vi "svfa_Conversion Utility (spectrum info).vi"(4 "spectral density desired":T1(ring), 5 "dx":dbl format="%.2f", 6 "desired scaling":T8 {"dB reference (0: no change)" format="%.2f"}, 7 "x0":dbl format="%.2f", 8 "error in (no error)":errorcluster, 10 "spectrum info in":T2={"channel name"="", "description"="", "x-axis units"=0, "spectral info"={"spectrum type"=enum."Power [Magnitude^2]", "linear/dB"=enum."linear", "window"=0, "window size"=0, "FFT size"=0}, "engineering units"=1, "custom label"="", "dB reference [EU]"=0.0, "peak units"=enum."rms", "weighting filter"=0, "spectral density?"=FALSE, "unit label"="", "spectrum skewed?"=FALSE, "complimentary spectrum units"=enum."none"} {"x-axis units" items=["Time (s)"=0, "Frequency-CB (Hz)"=1, "Frequency-CPB (Hz)"=1248, "Frequency-Arbitrary (Hz)"=2357, "Quefrency (s)"=2, "Revolutions (rev)"=3, "Order"=4, "Speed (RPM)"=11, "Speed (rad/s)"=21, "Index"=65535]; "weighting filter" items=["Linear", "A-weighting", "B-weighting", "C-weighting", "ITU-R 468-4", "Dolby", "CCITT", "C-message", "Wb", "Wc", "Wd", "We", "Wf", "Wh", "Wj", "Wk", "Wm", "AES17 20 kHz lowpass", "AES17 40 kHz lowpass", "AES17 20 kHz highpass", "AES17 40 kHz highpass"]; "dB reference [EU]" format="%.2f"; "engineering units" items=["custom..."=0, "V"=1, "A"=21, "C"=30, "pC"=31, "s"=32, "-"=29, "Pa"=2, "N"=20, "g"=3, "m/s^2"=4, "m/s"=5, "m"=6, "mm/s"=12, "mm"=13, "micron/s"=14, "micron"=15, "in/s^2"=7, "in/s"=8, "in"=9, "mil/s"=10, "mil"=11, "rad/s^2"=16, "rad/s"=17, "rad"=18, "deg/s^2"=26, "deg/s"=27, "deg"=28, "RPM"=22, "cycle/s^2"=23, "Hz"=24, "cycle"=25, "strain"=19]; "spectral info"."window" items=["None "=0, "Hanning"=1, "Hamming"=2, "Blackman-Harris"=3, "Exact Blackman"=4, "Blackman"=5, "Flat Top"=6, "4 Term B-Harris "=7, "7 Term B-Harris"=8, "Low Sidelobe"=9, "Force - Exponential"=10, "Gaussian"=62]}, 11 "input signal":dbl[](array[numeric]) format="%.2f") -> (0 "error out":errorcluster, 2 "spectrum info out":T2={"channel name"="", "description"="", "x-axis units"=0, "spectral info"={"spectrum type"=enum."Power [Magnitude^2]", "linear/dB"=enum."linear", "window"=0, "window size"=0, "FFT size"=0}, "engineering units"=1, "custom label"="", "dB reference [EU]"=0.0, "peak units"=enum."rms", "weighting filter"=0, "spectral density?"=FALSE, "unit label"="", "spectrum skewed?"=FALSE, "complimentary spectrum units"=enum."none"} {"x-axis units" items=["Time (s)"=0, "Frequency-CB (Hz)"=1, "Frequency-CPB (Hz)"=1248, "Frequency-Arbitrary (Hz)"=2357, "Quefrency (s)"=2, "Revolutions (rev)"=3, "Order"=4, "Speed (RPM)"=11, "Speed (rad/s)"=21, "Index"=65535]; "weighting filter" items=["Linear", "A-weighting", "B-weighting", "C-weighting", "ITU-R 468-4", "Dolby", "CCITT", "C-message", "Wb", "Wc", "Wd", "We", "Wf", "Wh", "Wj", "Wk", "Wm", "AES17 20 kHz lowpass", "AES17 40 kHz lowpass", "AES17 20 kHz highpass", "AES17 40 kHz highpass"]; "dB reference [EU]" format="%.2f"; "engineering units" items=["custom..."=0, "V"=1, "A"=21, "C"=30, "pC"=31, "s"=32, "-"=29, "Pa"=2, "N"=20, "g"=3, "m/s^2"=4, "m/s"=5, "m"=6, "mm/s"=12, "mm"=13, "micron/s"=14, "micron"=15, "in/s^2"=7, "in/s"=8, "in"=9, "mil/s"=10, "mil"=11, "rad/s^2"=16, "rad/s"=17, "rad"=18, "deg/s^2"=26, "deg/s"=27, "deg"=28, "RPM"=22, "cycle/s^2"=23, "Hz"=24, "cycle"=25, "strain"=19]; "spectral info"."window" items=["None "=0, "Hanning"=1, "Hamming"=2, "Blackman-Harris"=3, "Exact Blackman"=4, "Blackman"=5, "Flat Top"=6, "4 Term B-Harris "=7, "7 Term B-Harris"=8, "Low Sidelobe"=9, "Force - Exponential"=10, "Gaussian"=62]}, 3 "converted signal":dbl[](array[numeric]) format="%.2f")   [LabVIEW 2017]
uses:
  <vilib>/addons/_NISVFA/_Shared subVIs/Controls/svc_Spectrum Info.ctl
  <vilib>/addons/_NISVFA/_Shared subVIs/Controls/svc_X-Axis Units.ctl
  <vilib>/addons/_NISVFA/_Shared subVIs/Controls/svc_Spectrum Type.ctl
  <vilib>/addons/_NISVFA/_Shared subVIs/Controls/svc_Engineering Units Text Ring.ctl
  <vilib>/addons/_NISVFA/_Shared subVIs/Controls/svc_Weighting Filter Text Ring.ctl
  <vilib>/addons/_NISVFA/_Shared subVIs/Controls/svc_Complimentary Spectrum Units.ctl
  <vilib>/addons/_NISVFA/_Shared subVIs/Common/svc_Window Parameters.vi
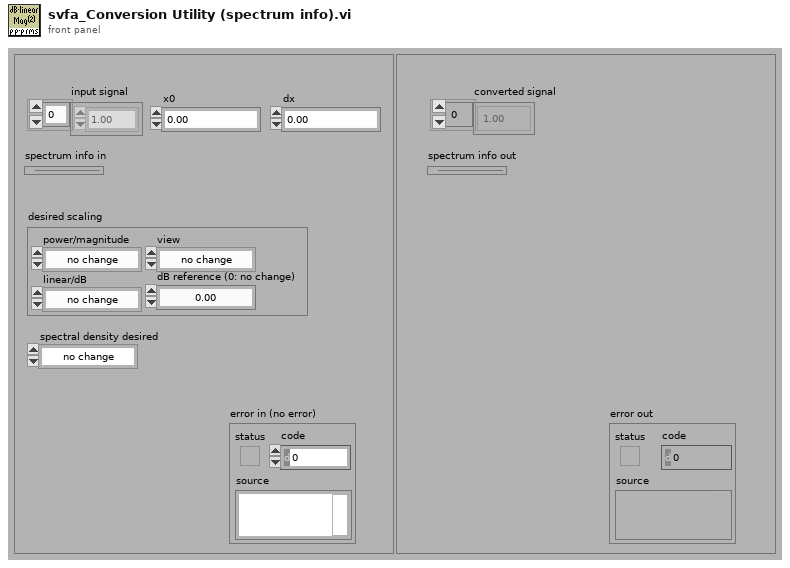
[diagram p1: front panel]
types:
  T1 = enum16{"no change", "spectrum", "spectral density"}
  T2 = typedef "svc_Spectrum Info.ctl" = cluster{"channel name":string, "description":string, "x-axis units":T3, "spectral info":cluster{"spectrum type":T4, "linear/dB":enum16{"linear", "dB"}, "window":u16, "window size":i32, "FFT size":i32}, "engineering units":T5, "custom label":string, "dB reference [EU]":dbl, "peak units":enum16{"rms", "peak", "peak-peak"}, "weighting filter":T6, "spectral density?":bool, "unit label":string, "spectrum skewed?":bool, "complimentary spectrum units":T7}
  T3 = typedef "svc_X-Axis Units.ctl" = u16
  T4 = typedef "svc_Spectrum Type.ctl" = enum16{"FFT Spectrum [complex]", "Amplitude [Magnitude]", "Power [Magnitude^2]", "Cross Spectrum [complex]", "Frequency Response [Complex]"}
  T5 = typedef "svc_Engineering Units Text Ring.ctl" = u16
  T6 = typedef "svc_Weighting Filter Text Ring.ctl" = u16
  T7 = typedef "svc_Complimentary Spectrum Units.ctl" = enum16{"none", "radians", "degrees", "cycles", "imaginary"}
  T8 = cluster{"linear/dB":enum16{"no change", "linear", "dB"}, "dB reference (0: no change)":dbl, "power/magnitude":enum16{"no change", "power", "magnitude"}, "view":enum16{"no change", "rms", "peak", "peak-peak"}}
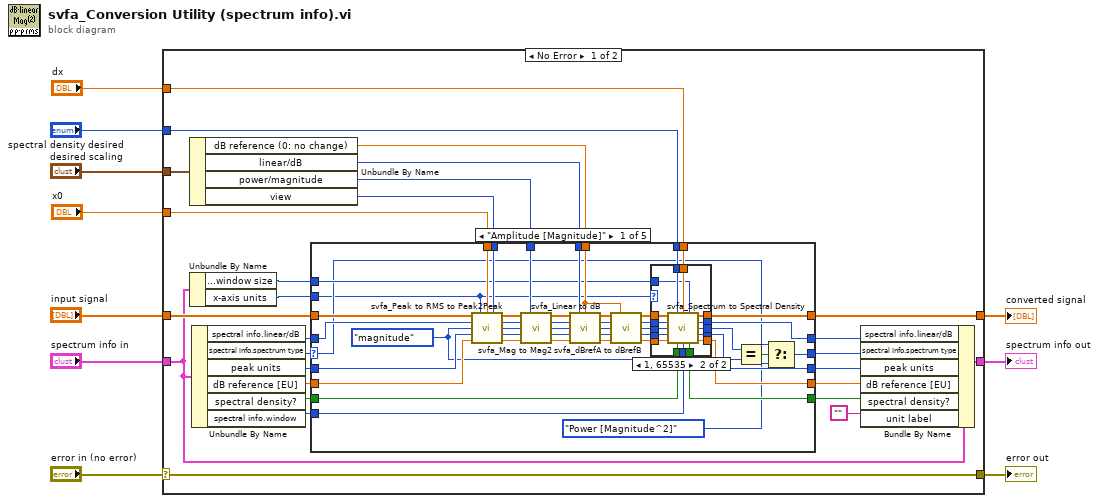
[diagram p0: block diagram]
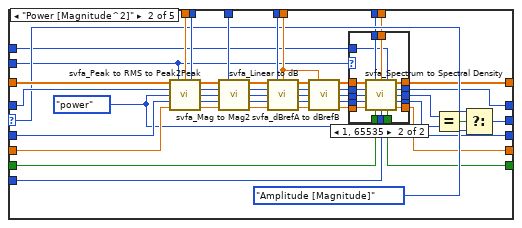
[diagram p3: hidden frame]
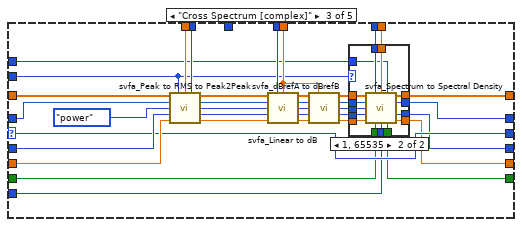
[diagram p5: hidden frame]
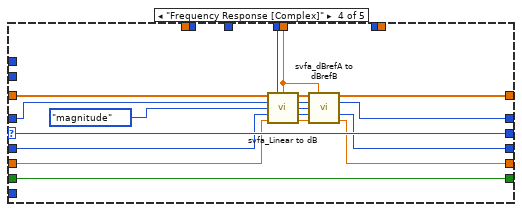
[diagram p7: hidden frame]
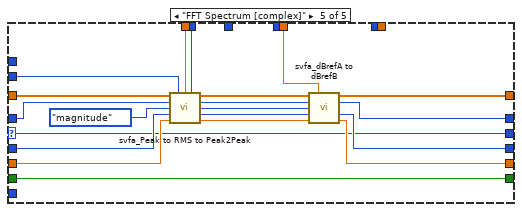
[diagram p8: hidden frame]
diagram:
  n1 = case shown="No Error" "error in (no error)" {
    selector: "error in (no error)" -> [w36 w268]
    tunnel: "input signal" -> [w33 w270]
    tunnel: [w20 w270] -> w4
    tunnel: "desired scaling" -> [w37 _]
    tunnel: "spectrum info in" -> [w16 w269]
    tunnel: [w26 w269] -> w7
    tunnel: [w36 w268] -> w5
    tunnel: "x0" -> [w31 _]
    tunnel: "spectral density desired" -> [w25 _]
    tunnel: "dx" -> [w24 _]
    frame No Error {
      n2 = Unbundle By Name(w37) -> ("dB reference (0: no change)"=w30:dbl, "linear/dB"=w35:enum16{"no change", "linear", "dB"}, "power/magnitude"=w34:enum16{"no change", "power", "magnitude"}, "view"=w32:enum16{"no change", "rms", "peak", "peak-peak"})
      n3 = Unbundle By Name(w16) -> ("spectral info.window size"=w14:i32, "x-axis units"=w15:T3)
      n4 = Unbundle By Name(w16) -> ("spectral info.linear/dB"=w28:enum16{"linear", "dB"}, "spectral info.spectrum type"=w12:T4, "peak units"=w13:enum16{"rms", "peak", "peak-peak"}, "dB reference [EU]"=w29:dbl, "spectral density?"=w23:bool, "spectral info.window"=w22:u16)
      n5 = case shown="\"Amplitude [Magnitude]\"" w12 {
        selector: w12 -> [w40 w124 w190 w240 w248]
        tunnel: w35 -> [w83 w151 w209 w247 _]
        tunnel: w34 -> [w82 w150 _ _ _]
        tunnel: w33 -> [w81 w149 w208 w237 w267]
        tunnel: w32 -> [w77 w145 w206 _ w266]
        tunnel: w31 -> [w67 w135 w202 _ w265]
        tunnel: w30 -> [w64 w132 w201 w242 w264]
        tunnel: w29 -> [w62 w130 w199 w234 w263]
        tunnel: w28 -> [w61 w129 w198 w236 w262]
        tunnel: [w59 w127 w190 w240 w248] -> w27
        tunnel: w25 -> [w58 w107 w186 _ _]
        tunnel: w24 -> [w57 w106 w185 _ _]
        tunnel: w23 -> [w56 w114 w176 w232 w251]
        tunnel: w22 -> [w55 w113 w175 _ _]
        tunnel: [w54 w112 w174 w232 w251] -> w21
        tunnel: [w48 w122 w177 w239 w253] -> w20
        tunnel: [w47 w108 w178 w238 w252] -> w19
        tunnel: [w46 w110 w179 w230 w249] -> w18
        tunnel: [w45 w109 w180 w233 w250] -> w17
        tunnel: w15 -> [w38 w121 w187 _ w261]
        tunnel: w14 -> [w44 w120 w188 _ _]
        tunnel: w13 -> [w43 w126 w197 w231 w260]
        frame "Amplitude [Magnitude]" {
          w42 = enum16{"power", "magnitude"}."magnitude" ("power/magnitude")
          n6 = call <vilib>:"svfa_Peak to RMS to Peak2Peak.vi"("input signal"=w81, "x-axis units"=w38, "x0"=w67, "view desired"=w77, "linear/dB"=w61, "power/magnitude"=w42, "view in"=w43, "dB reference"=w62) -> ("scale converted signal"=w80:dbl[], "linear/dB (dupl)"=w76:enum16{"linear", "dB"}, "power/magnitude (dupl)"=w66:enum16{"power", "magnitude"}, "view out"=w73:enum16{"rms", "peak", "peak-peak"}, "dB reference (dupl)"=w72:dbl)  [unwired: 3 in]
          n7 = call <vilib>:"svfa_Mag to Mag2.vi"("input signal"=w80, "power/magnitude desired"=w82, "linear/dB"=w76, "power/magnitude"=w66, "view"=w73, "dB reference"=w72) -> ("converted signal"=w79:dbl[], "dup linear/dB"=w75:enum16{"linear", "dB"}, "power/magnitude (out)"=w65:enum16{"power", "magnitude"}, "dup view"=w70:enum16{"rms", "peak", "peak-peak"}, "dB reference (out)"=w71:dbl)  [unwired: 5 in]
          n8 = call <vilib>:"svfa_Linear to dB.vi"("input signal"=w79, "linear/dB desired"=w83, "dB reference (desired)"=w64, "linear/dB (in)"=w75, "power/magnitude"=w65, "view in"=w70, "dB reference"=w71) -> ("converted signal"=w78:dbl[], "linear/dB (out)"=w74:enum16{"linear", "dB"}, "power/magnitude (dupl)"=w63:enum16{"power", "magnitude"}, "view out"=w69:enum16{"rms", "peak", "peak-peak"}, "dB reference (dupl)"=w68:dbl)  [unwired: 4 in]
          n9 = call <vilib>:"svfa_dBrefA to dBrefB.vi"("input signal"=w78, "dB reference (desired)"=w64, "linear/dB"=w74, "power/magnitude"=w63, "view"=w69, "dB reference"=w68) -> ("converted signal"=w49:dbl[], "linear/dB (dupl)"=w50:enum16{"linear", "dB"}, "power/magnitude (dupl)"=w51:enum16{"power", "magnitude"}, "dup view"=w52:enum16{"rms", "peak", "peak-peak"}, "dB reference (out)"=w53:dbl)  [unwired: 5 in]
          n10 = case shown="1, 65535" w38 {
            tunnel: w58 -> [_ w105]
            tunnel: w57 -> [_ w104]
            tunnel: w56 -> [w84 w103]
            tunnel: w55 -> [_ w102]
            tunnel: [w84 w101] -> w54
            tunnel: w53 -> [w85 w100]
            tunnel: w52 -> [w86 w99]
            tunnel: w51 -> [w87 w98]
            tunnel: w50 -> [w88 w97]
            tunnel: w49 -> [w89 w96]
            tunnel: [w89 w95] -> w48
            tunnel: [w88 w94] -> w47
            tunnel: [w86 w93] -> w46
            tunnel: [w85 w92] -> w45
            tunnel: w44 -> [_ w91]
            tunnel: [w87 w90] -> w41
            frame Default {
            }
            frame 1, 65535 {
              n11 = call <vilib>:"svfa_Spectrum to Spectral Density.vi"("input signal"=w96, "spectral density desired"=w105, "df"=w104, "window size"=w91, "linear/dB"=w97, "power/magnitude"=w98, "view"=w99, "dB reference"=w100, "spectral density?"=w103, "window"=w102) -> ("converted signal"=w95:dbl[], "dup linear/dB"=w94:enum16{"linear", "dB"}, "power/magnitude (dupl)"=w90:enum16{"power", "magnitude"}, "dup view"=w93:enum16{"rms", "peak", "peak-peak"}, "spectral density?"=w101:bool, "dB reference (out)"=w92:dbl)
            }
          }
          n12 = Equal?(x=w41, y=w42) -> (x = y?=w60:bool)
          n13 = Select(t=w40, s=w60, f=svc_Spectrum_Type."Power [Magnitude^2]" ("spectral info.spectrum type")) -> (s? t:f=w59:T4)
        }
        frame "Power [Magnitude^2]" {
          w125 = enum16{"power", "magnitude"}."power" ("power/magnitude")
          n14 = call <vilib>:"svfa_Peak to RMS to Peak2Peak.vi"("input signal"=w149, "x-axis units"=w121, "x0"=w135, "view desired"=w145, "linear/dB"=w129, "power/magnitude"=w125, "view in"=w126, "dB reference"=w130) -> ("scale converted signal"=w148:dbl[], "linear/dB (dupl)"=w144:enum16{"linear", "dB"}, "power/magnitude (dupl)"=w134:enum16{"power", "magnitude"}, "view out"=w141:enum16{"rms", "peak", "peak-peak"}, "dB reference (dupl)"=w140:dbl)  [unwired: 3 in]
          n15 = call <vilib>:"svfa_Mag to Mag2.vi"("input signal"=w148, "power/magnitude desired"=w150, "linear/dB"=w144, "power/magnitude"=w134, "view"=w141, "dB reference"=w140) -> ("converted signal"=w147:dbl[], "dup linear/dB"=w143:enum16{"linear", "dB"}, "power/magnitude (out)"=w133:enum16{"power", "magnitude"}, "dup view"=w138:enum16{"rms", "peak", "peak-peak"}, "dB reference (out)"=w139:dbl)  [unwired: 5 in]
          n16 = call <vilib>:"svfa_Linear to dB.vi"("input signal"=w147, "linear/dB desired"=w151, "dB reference (desired)"=w132, "linear/dB (in)"=w143, "power/magnitude"=w133, "view in"=w138, "dB reference"=w139) -> ("converted signal"=w146:dbl[], "linear/dB (out)"=w142:enum16{"linear", "dB"}, "power/magnitude (dupl)"=w131:enum16{"power", "magnitude"}, "view out"=w137:enum16{"rms", "peak", "peak-peak"}, "dB reference (dupl)"=w136:dbl)  [unwired: 4 in]
          n17 = call <vilib>:"svfa_dBrefA to dBrefB.vi"("input signal"=w146, "dB reference (desired)"=w132, "linear/dB"=w142, "power/magnitude"=w131, "view"=w137, "dB reference"=w136) -> ("converted signal"=w119:dbl[], "linear/dB (dupl)"=w118:enum16{"linear", "dB"}, "power/magnitude (dupl)"=w117:enum16{"power", "magnitude"}, "dup view"=w116:enum16{"rms", "peak", "peak-peak"}, "dB reference (out)"=w115:dbl)  [unwired: 5 in]
          n18 = case shown="1, 65535" w121 {
            tunnel: w107 -> [_ w173]
            tunnel: w106 -> [_ w172]
            tunnel: w114 -> [w152 w171]
            tunnel: w113 -> [_ w170]
            tunnel: [w152 w169] -> w112
            tunnel: w115 -> [w153 w168]
            tunnel: w116 -> [w154 w167]
            tunnel: w117 -> [w155 w166]
            tunnel: w118 -> [w156 w165]
            tunnel: w119 -> [w157 w164]
            tunnel: [w157 w163] -> w122
            tunnel: [w156 w162] -> w108
            tunnel: [w154 w161] -> w110
            tunnel: [w153 w160] -> w109
            tunnel: w120 -> [_ w159]
            tunnel: [w155 w158] -> w111
            frame Default {
            }
            frame 1, 65535 {
              n19 = call <vilib>:"svfa_Spectrum to Spectral Density.vi"("input signal"=w164, "spectral density desired"=w173, "df"=w172, "window size"=w159, "linear/dB"=w165, "power/magnitude"=w166, "view"=w167, "dB reference"=w168, "spectral density?"=w171, "window"=w170) -> ("converted signal"=w163:dbl[], "dup linear/dB"=w162:enum16{"linear", "dB"}, "power/magnitude (dupl)"=w158:enum16{"power", "magnitude"}, "dup view"=w161:enum16{"rms", "peak", "peak-peak"}, "spectral density?"=w169:bool, "dB reference (out)"=w160:dbl)
            }
          }
          n20 = Equal?(x=w111, y=w125) -> (x = y?=w128:bool)
          n21 = Select(t=w124, s=w128, f=svc_Spectrum_Type."Amplitude [Magnitude]" ("spectral info.spectrum type")) -> (s? t:f=w127:T4)
        }
        frame "Cross Spectrum [complex]" {
          n22 = call <vilib>:"svfa_Peak to RMS to Peak2Peak.vi"("input signal"=w208, "x-axis units"=w187, "x0"=w202, "view desired"=w206, "linear/dB"=w198, "power/magnitude"=enum16{"power", "magnitude"}."power", "view in"=w197, "dB reference"=w199) -> ("scale converted signal"=w195:dbl[], "linear/dB (dupl)"=w194:enum16{"linear", "dB"}, "power/magnitude (dupl)"=w193:enum16{"power", "magnitude"}, "view out"=w192:enum16{"rms", "peak", "peak-peak"}, "dB reference (dupl)"=w191:dbl)  [unwired: 3 in]
          n23 = call <vilib>:"svfa_Linear to dB.vi"("input signal"=w195, "linear/dB desired"=w209, "dB reference (desired)"=w201, "linear/dB (in)"=w194, "power/magnitude"=w193, "view in"=w192, "dB reference"=w191) -> ("converted signal"=w207:dbl[], "linear/dB (out)"=w205:enum16{"linear", "dB"}, "power/magnitude (dupl)"=w200:enum16{"power", "magnitude"}, "view out"=w204:enum16{"rms", "peak", "peak-peak"}, "dB reference (dupl)"=w203:dbl)  [unwired: 4 in]
          n24 = call <vilib>:"svfa_dBrefA to dBrefB.vi"("input signal"=w207, "dB reference (desired)"=w201, "linear/dB"=w205, "power/magnitude"=w200, "view"=w204, "dB reference"=w203) -> ("converted signal"=w189:dbl[], "linear/dB (dupl)"=w184:enum16{"linear", "dB"}, "power/magnitude (dupl)"=w183:enum16{"power", "magnitude"}, "dup view"=w182:enum16{"rms", "peak", "peak-peak"}, "dB reference (out)"=w181:dbl)  [unwired: 5 in]
          n25 = case shown="1, 65535" w187 {
            tunnel: w186 -> [_ w229]
            tunnel: w185 -> [_ w228]
            tunnel: w176 -> [w210 w227]
            tunnel: w175 -> [_ w226]
            tunnel: [w210 w225] -> w174
            tunnel: w181 -> [w211 w224]
            tunnel: w182 -> [w212 w223]
            tunnel: w183 -> [_ w222]
            tunnel: w184 -> [w213 w221]
            tunnel: w189 -> [w214 w220]
            tunnel: [w214 w219] -> w177
            tunnel: [w213 w218] -> w178
            tunnel: [w212 w217] -> w179
            tunnel: [w211 w216] -> w180
            tunnel: w188 -> [_ w215]
            frame Default {
            }
            frame 1, 65535 {
              n26 = call <vilib>:"svfa_Spectrum to Spectral Density.vi"("input signal"=w220, "spectral density desired"=w229, "df"=w228, "window size"=w215, "linear/dB"=w221, "power/magnitude"=w222, "view"=w223, "dB reference"=w224, "spectral density?"=w227, "window"=w226) -> ("converted signal"=w219:dbl[], "dup linear/dB"=w218:enum16{"linear", "dB"}, "dup view"=w217:enum16{"rms", "peak", "peak-peak"}, "spectral density?"=w225:bool, "dB reference (out)"=w216:dbl)  [unwired: 1 out]
            }
          }
        }
        frame "Frequency Response [Complex]" {
          n27 = call <vilib>:"svfa_Linear to dB.vi"("input signal"=w237, "linear/dB desired"=w247, "dB reference (desired)"=w242, "linear/dB (in)"=w236, "power/magnitude"=enum16{"power", "magnitude"}."magnitude", "view in"=w231, "dB reference"=w234) -> ("converted signal"=w246:dbl[], "linear/dB (out)"=w245:enum16{"linear", "dB"}, "power/magnitude (dupl)"=w241:enum16{"power", "magnitude"}, "view out"=w244:enum16{"rms", "peak", "peak-peak"}, "dB reference (dupl)"=w243:dbl)  [unwired: 4 in]
          n28 = call <vilib>:"svfa_dBrefA to dBrefB.vi"("input signal"=w246, "dB reference (desired)"=w242, "linear/dB"=w245, "power/magnitude"=w241, "view"=w244, "dB reference"=w243) -> ("converted signal"=w239:dbl[], "linear/dB (dupl)"=w238:enum16{"linear", "dB"}, "dup view"=w230:enum16{"rms", "peak", "peak-peak"}, "dB reference (out)"=w233:dbl)  [unwired: 5 in, 1 out]
        }
        frame "FFT Spectrum [complex]" {
          n29 = call <vilib>:"svfa_Peak to RMS to Peak2Peak.vi"("input signal"=w267, "x-axis units"=w261, "x0"=w265, "view desired"=w266, "linear/dB"=w262, "power/magnitude"=enum16{"power", "magnitude"}."magnitude", "view in"=w260, "dB reference"=w263) -> ("scale converted signal"=w258:dbl[], "linear/dB (dupl)"=w257:enum16{"linear", "dB"}, "power/magnitude (dupl)"=w256:enum16{"power", "magnitude"}, "view out"=w255:enum16{"rms", "peak", "peak-peak"}, "dB reference (dupl)"=w254:dbl)  [unwired: 3 in]
          n30 = call <vilib>:"svfa_dBrefA to dBrefB.vi"("input signal"=w258, "dB reference (desired)"=w264, "linear/dB"=w257, "power/magnitude"=w256, "view"=w255, "dB reference"=w254) -> ("converted signal"=w253:dbl[], "linear/dB (dupl)"=w252:enum16{"linear", "dB"}, "dup view"=w249:enum16{"rms", "peak", "peak-peak"}, "dB reference (out)"=w250:dbl)  [unwired: 5 in, 1 out]
        }
      }
      n31 = Bundle By Name(cluster=w16, "spectral info.linear/dB"=w19, "spectral info.spectrum type"=w27, "peak units"=w18, "dB reference [EU]"=w17, "spectral density?"=w21, "unit label"="") -> (w26:T2)
    }
    frame Error {
    }
  }
  "spectrum info out" <- w7
  "error out" <- w5
  "converted signal" <- w4
